vi "DI Port Num Pins.vi"() -> ()   [LabVIEW 2011, in "LabVIEW Interface for ChipKit.lvlib"]
uses:
  LabVIEW Interface for ChipKit.lvlib
panel:
  in  "DI Port Num Pins":i32
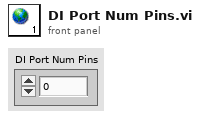
[diagram p1: front panel]
diagram:
